vi "LHF.DB.Mongo.Collection.Core.Aggregate.vi"(6 "Extract ObjectID":bool, 8 "error in (no error)":errorcluster, 9 "Collection":string, 10 "operations":refnum<k24>[](array[refnum]), 11 "LHF.DB.Mongo in":refnum<class "LHF.DB.Mongo.lvclass">) -> (0 "error out":errorcluster, 1 "Documents":string[](array[string]), 2 "operations out":refnum<k24>[](array[refnum]), 3 "LHF.DB.Mongo out":refnum<class "LHF.DB.Mongo.lvclass">, 5 "ObjectID":string[](array[string]))   [LabVIEW 2013, in "LHF.DB.Mongo.lvclass"]
uses:
  LHF.DB.Mongo.lvclass
  C:/Users/schim/Desktop/Projetos/LabVIEW-MongoDB/src/Driver/MongoDB.Bson.dll
  Driver/MongoDB.Bson.dll
  C:/Users/schim/Desktop/Projetos/LabVIEW-MongoDB/src/Driver/MongoDB.Driver.dll
  Driver/MongoDB.Driver.dll
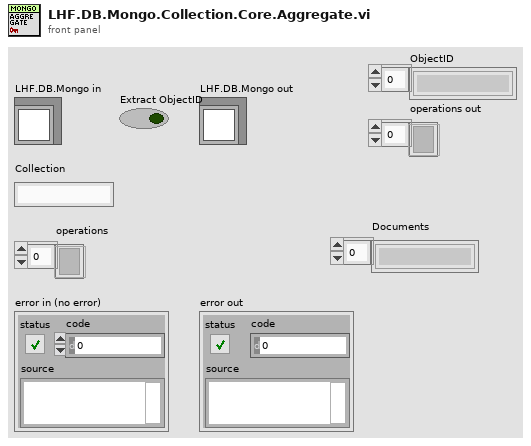
[diagram p1: front panel]
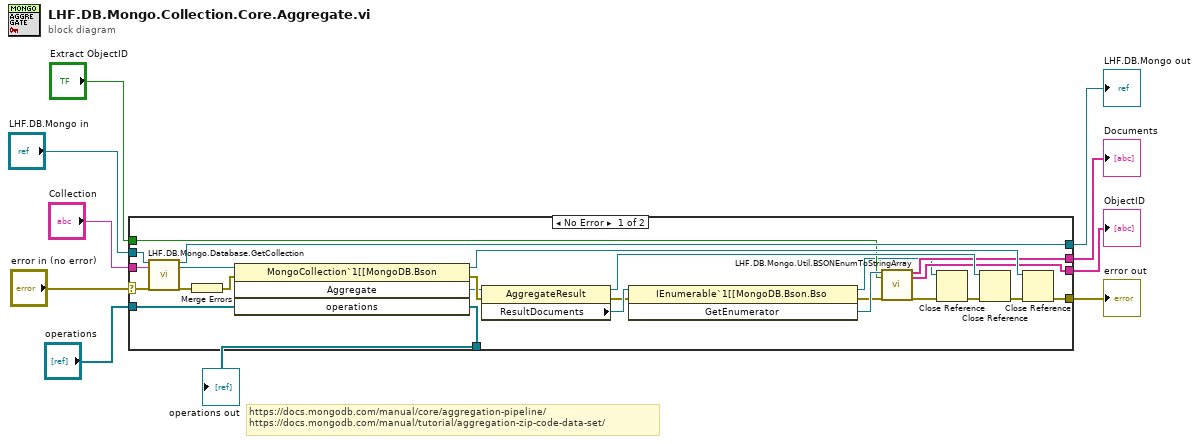
[diagram p0: block diagram]
diagram:
  # "https://docs.mongodb.com/manual/core/aggregation-pipeline/\nhttps://docs.mongodb.com/manual/tutorial/aggregation-zip-code-data-set/"
  n1 = case shown="No Error" "error in (no error)" {
    selector: "error in (no error)" -> [w17 w38]
    tunnel: "operations" -> [w35 w36]
    tunnel: "LHF.DB.Mongo in" -> [w26 w37]
    tunnel: [w25 w37] -> w8
    tunnel: "Collection" -> [w24 _]
    tunnel: [w20 _] -> w6
    tunnel: [w18 w38] -> w5
    tunnel: [w16 _] -> w3
    tunnel: "Extract ObjectID" -> [w15 _]
    tunnel: [w11 w36] -> w1
    frame No Error {
      n2 = call "LHF.DB.Mongo.Database.GetCollection.vi"("LHF.DB.Mongo in"=w26, "collectionName"=w24, "error in (no error)"=w17) -> ("LHF.DB.Mongo in"=w25:refnum<class "LHF.DB.Mongo.lvclass">, "MongoCollection"=w28:refnum<k24>, "error out"=w29:errorcluster)  [unwired: 14 in]
      n3 = Merge Errors(w29) -> (w30:errorcluster)
      n4 = invoke class="MongoCollection`1[[MongoDB.Bson" method="Aggregate"(reference=w28, error in=w30, "operations"=w35) -> (reference out=w34:refnum<k24>, error out=w31:errorcluster, "Aggregate"=w27:refnum<k24>, "operations"=w11:refnum<k24>[])  [unwired: 1 in]
      n5 = property class="AggregateResult"(reference=w27, error in=w31) -> (reference out=w32:refnum<k24>, error out=w19:errorcluster, "ResultDocuments"=w23:refnum<k24>)
      n6 = invoke class="IEnumerable`1[[MongoDB.Bson.Bso" method="GetEnumerator"(reference=w23, error in=w19) -> (reference out=w14:refnum<k24>, error out=w21:errorcluster, "GetEnumerator"=w22:refnum<k24>)  [unwired: 1 in]
      n7 = call "LHF.DB.Mongo.Util.BSONEnumToStringArray.vi"("BsonENUM"=w22, "Extract ObjectID"=w15, "error in (no error)"=w21) -> ("Documents"=w20:string[], "ObjectIDs"=w16:string[], "error out"=w13:errorcluster)  [unwired: 14 in]
      n8 = Close Reference(reference=w14, error in (no error)=w13) -> (error out=w12:errorcluster)
      n9 = Close Reference(reference=w32, error in (no error)=w12) -> (error out=w33:errorcluster)
      n10 = Close Reference(reference=w34, error in (no error)=w33) -> (error out=w18:errorcluster)
    }
    frame Error {
    }
  }
  "error out" <- w5
  "Documents" <- w6
  "LHF.DB.Mongo out" <- w8
  "ObjectID" <- w3
  "operations out" <- w1
